vi "Write focusName.vi"(8 "error in (no error)":errorcluster, 10 "focusName":T1, 11 "FocusSelect in":refnum<class "FocusSelect.lvclass">) -> (0 "error out":errorcluster, 3 "FocusSelect out":refnum<class "FocusSelect.lvclass">)   [LabVIEW 2014, in "TCSDataDefinitions.lvlib" / "TCSCommand.lvlib" / "FocusSelect.lvclass"]
uses:
  FocusSelect.lvclass
  Enumerations/FocusNameTypes.ctl
  FocusSelect.lvclass/FocusSelect.ctl
  TCSCommand.lvlib
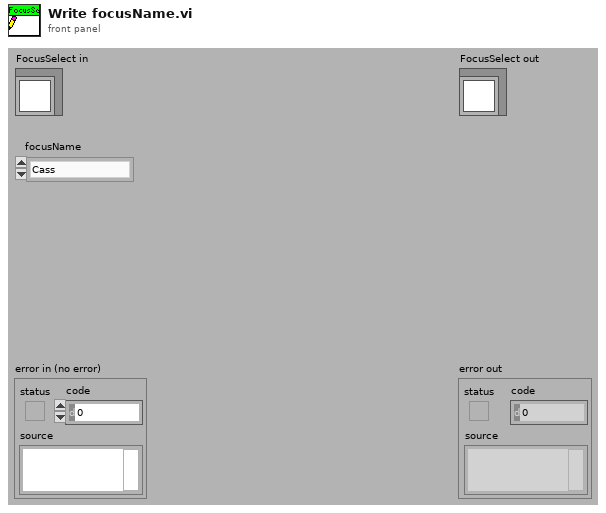
[diagram p1: front panel]
types:
  T1 = typedef "TCSDataDefinitions.lvlib/TCSCommand.lvlib/FocusNameTypes.ctl" = enum16{"Cass", "Prime", "Nasmyth1", "Nasmyth2", "BentCass1", "BentCass2", "BentCass3", "BentCass4", "BentCass5", "BentCass6"}
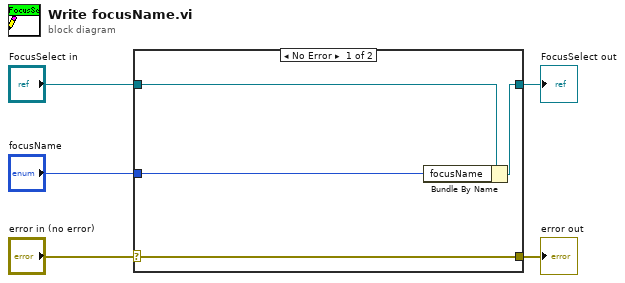
[diagram p0: block diagram]
diagram:
  n1 = case shown="No Error" "error in (no error)" {
    selector: "error in (no error)" -> [w9 w10]
    tunnel: [w9 w10] -> w4
    tunnel: [w7 w11] -> w2
    tunnel: "FocusSelect in" -> [w8 w11]
    tunnel: "focusName" -> [w6 _]
    frame No Error {
      n2 = Bundle By Name(cluster=w8, "focusName"=w6) -> (w7:refnum<class "FocusSelect.lvclass">)
    }
    frame Error {
    }
  }
  "error out" <- w4
  "FocusSelect out" <- w2
